vi "Finish.vi"(8 "error in (no error)":errorcluster) -> ()   [LabVIEW 2013]
uses:
  <vilib>/ActorFramework/Stop Msg/Stop Msg.lvclass/Stop Msg.ctl
  <vilib>/ActorFramework/Message Enqueuer/Message Enqueuer.lvclass/Message Enqueuer.ctl
  <vilib>/ActorFramework/Message Enqueuer/Enqueue Critical.vi
  Robot Global.vi
  <vilib>/ActorFramework/Message Priority Queue/Priority Enqueue.vi
  <vilib>/ActorFramework/Message Enqueuer/Message Enqueuer.lvclass
  <vilib>/ActorFramework/Stop Msg/Stop Msg.lvclass
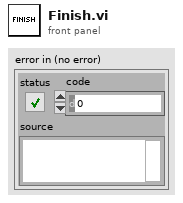
[diagram p1: front panel]
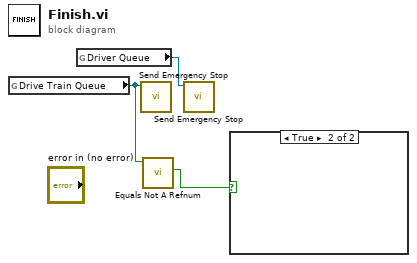
[diagram p0: block diagram]
diagram:
  n1 = global read "Robot Global.vi" "Drive Train Queue"() -> (w2:refnum<class "Message Enqueuer.lvclass">)
  n2 = global read "Robot Global.vi" "Driver Queue"() -> (w3:refnum<class "Message Enqueuer.lvclass">)
  n3 = call <vilib>:"Send Emergency Stop.vi"("Message Enqueuer"=w2) -> ()  [unwired: 10 in, 1 out]
  n4 = call <vilib>:"Equals Not A Refnum.vi"("Message Enqueuer"=w2) -> ("Not a refnum?"=w1:bool)  [unwired: 10 in]
  n5 = call <vilib>:"Send Emergency Stop.vi"("Message Enqueuer"=w3) -> ()  [unwired: 10 in, 1 out]
  n6 = case shown="True" w1 {
    frame False {
    }
    frame True {
    }
  }
